vi "BDR_Report.vi"(8 "error in (no error)":errorcluster, 11 "Ref In":T1={"MS SQL Connection"=refnum, "UDL File"=path "", "Time"="", "DCODE"="", "WIP+1"=0, "MC No?"=0, "POKAYOKE?"=FALSE, "Expected Result"="", "Result [Status]"="", "Clock"=0.0, "RFID"="", "WIP Queue"=refnum, "TS Parameter"={"ProfitCenterCode"="", "LineCode"="", "WorkOrderNumber"="", "Model"="", "Model_with_Prefix"="", "VendorCode"="", "SetParameterDateCode"="", "PokaYoke"=0, "Target"=1, "Live_DateCode"="", "CustomerPartNumber"="", "Hand"="", "sBarcode"=FALSE, "FCA"=0, "Ent_Stamp"=timestamp(0 s since 1904-01-01), "STS_CD"=0.0}, "Data_Queue"=[], "RFID Serial No."=""} {"TS Parameter"."FCA" format="%01d"; "TS Parameter"."Target" min=1 max=100000; "TS Parameter"."PokaYoke" min=0 max=1}) -> (0 "error out":errorcluster)   [LabVIEW 2020]
uses:
  Controls/TD SQL.ctl
  <vilib>/addons/database/Connection.llb/Conn ObjectReference.ctl
  Controls/WIP_State.ctl
  Controls/TS_Parameter.ctl
  <vilib>/addons/database/Connection.llb/Conn Execute.vi
  <vilib>/addons/database/Recordset.llb/Rec Fetch Recordset Data (R).vi
  <vilib>/addons/database/Recordset.llb/Rec Destroy - Connection.vi
  <vilib>/addons/database/_DB Variant To Data/Database Variant To Data.xnode
  <vilib>/addons/database/NI_Database_API.lvlib
panel:
  in  "Exit":bool
  in  "Report":i32(listbox)
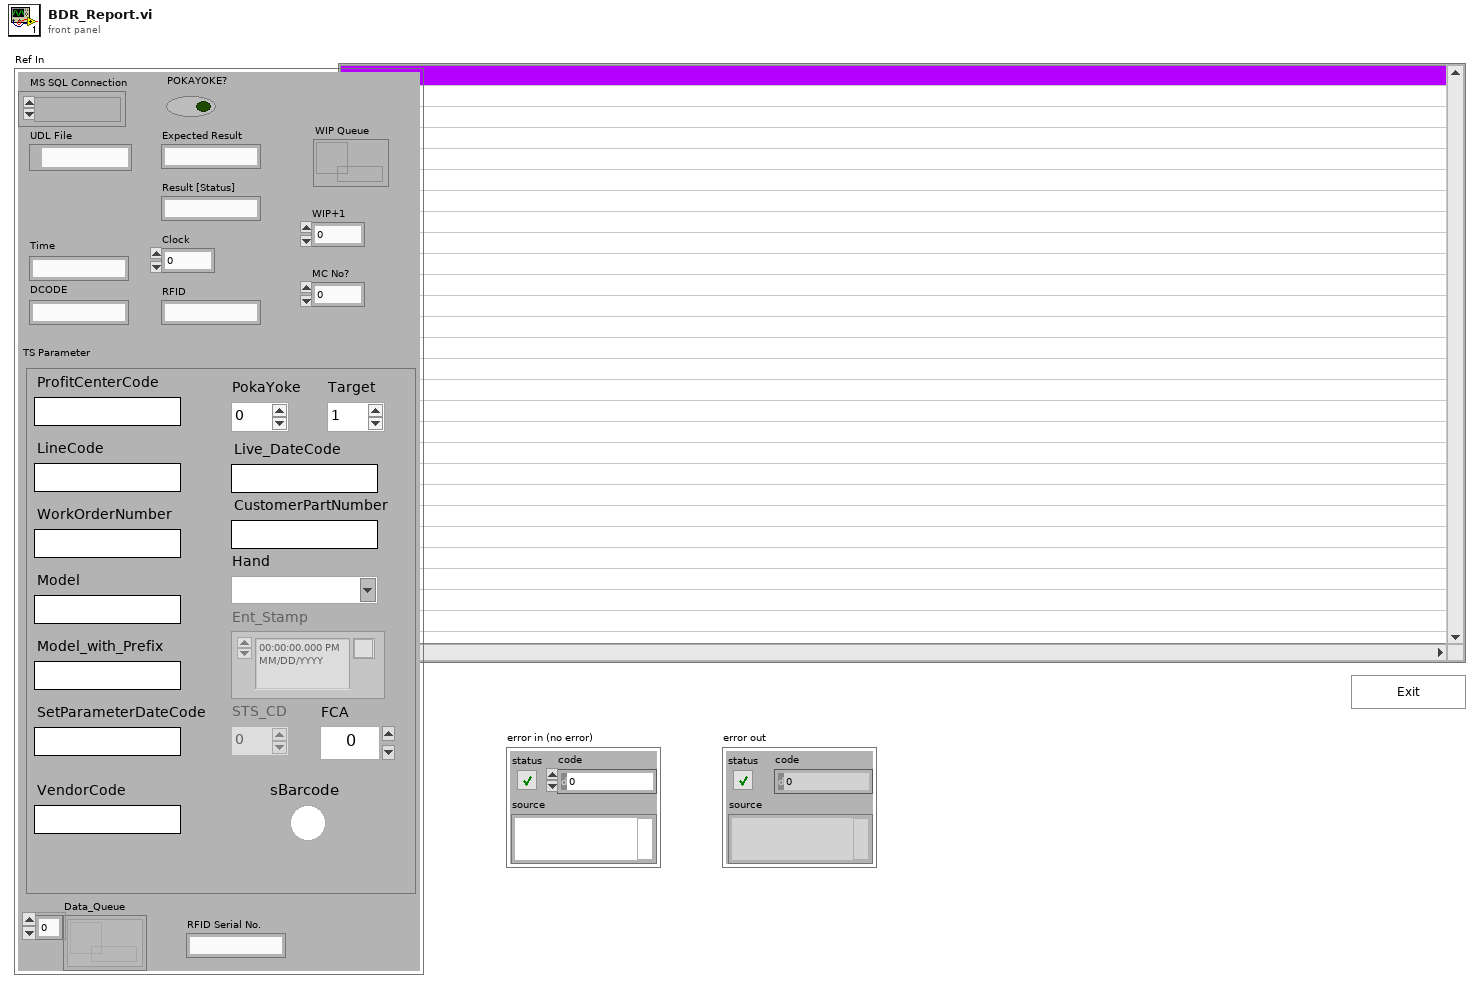
[diagram p1: front panel]
types:
  T1 = typedef "TD SQL.ctl" = cluster{"MS SQL Connection":T2, "UDL File":path, "Time":string, "DCODE":string, "WIP+1":i64, "MC No?":i32, "POKAYOKE?":bool, "Expected Result":string, "Result [Status]":string, "Clock":dbl, "RFID":string, "WIP Queue":refnum<queue>, "TS Parameter":T3, "Data_Queue":refnum<queue>[], "RFID Serial No.":string}
  T2 = typedef "NI_Database_API.lvlib/Conn ObjectReference.ctl" = refnum<k1>
  T3 = typedef "TS_Parameter.ctl" = cluster{"ProfitCenterCode":string, "LineCode":string, "WorkOrderNumber":string, "Model":string, "Model_with_Prefix":string, "VendorCode":string, "SetParameterDateCode":string, "PokaYoke":i32, "Target":i32, "Live_DateCode":string, "CustomerPartNumber":string, "Hand":string, "sBarcode":bool, "FCA":i32, "Ent_Stamp":timestamp, "STS_CD":dbl}
  T4 = typedef "NI_Database_API.lvlib/Rec ObjectReference.ctl" = refnum<k1>
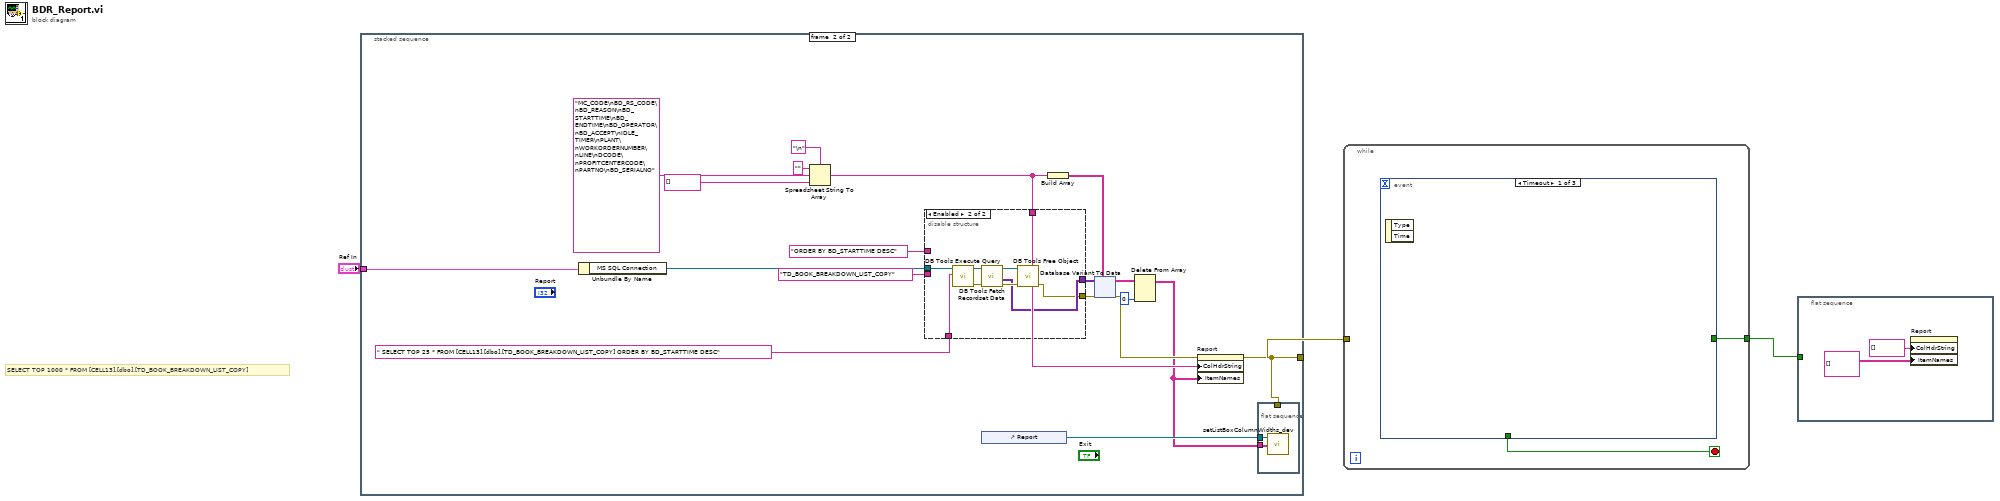
[diagram p0: block diagram]
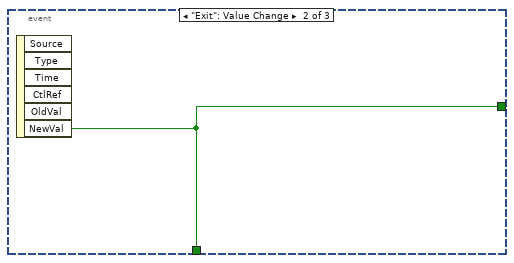
[diagram p2: hidden frame]
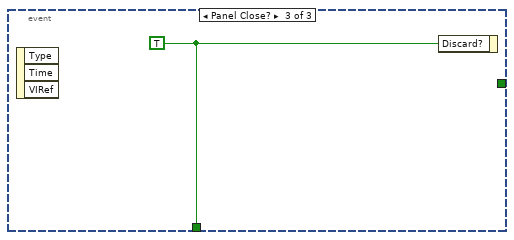
[diagram p3: hidden frame]
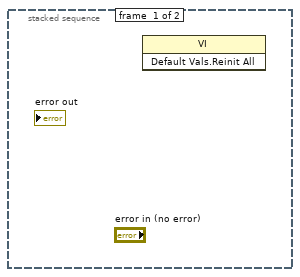
[diagram p4: hidden frame]
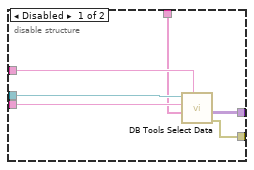
[diagram p5: hidden frame]
diagram:
  # "SELECT TOP 1000 * FROM [CELL13].[dbo].[TD_BOOK_BREAKDOWN_LIST_COPY]"
  n1 = stacked-sequence {
    tunnel: "Ref In" -> [_ w8]
    tunnel: [_ w9] -> w3
    frame #0 {
      n2 = invoke class="VI" method="Default Vals.Reinit All"() -> ()  [unwired: 3 in, 3 out]
    }
    frame #1 {
      n3 = Unbundle By Name(w8) -> ("MS SQL Connection"=w22:T2)
      n4 = Spreadsheet String To Array(delimiter (Tab)="\n", format string="", spreadsheet string="MC_CODE\nBD_RS_CODE\nBD_REASON\nBD_STARTTIME\nBD_ENDTIME\nBD_OPERATOR\nBD_ACCEPT\nIDLE_TIMER\nPLANT\nWORKORDERNUMBER\nLINE\nDCODE\nPROFITCENTERCODE\nPARTNO\nBD_SERIALNO", array type (2D Dbl)=string[] []) -> (array=w13:string[])
      n5 = disable-structure shown="Enabled" {
        disable-tunnel: w22 -> [w28 w32]
        disable-tunnel: "TD_BOOK_BREAKDOWN_LIST_COPY" ("table") -> [w27 _]
        disable-tunnel: [w26 w31] -> w16
        disable-tunnel: "ORDER BY BD_STARTTIME DESC" ("condition") -> [w25 _]
        disable-tunnel: w13 -> [w24 _]
        disable-tunnel: [w23 w29] -> w11
        disable-tunnel: " SELECT TOP 25 * FROM [CELL13].[dbo].[TD_BOOK_BREAKDOWN_LIST_COPY] ORDER BY BD_STARTTIME DESC" ("condition") -> [_ w30]
        frame Disabled {
          n6 = call <vilib>:"DB Tools Select Data.vi"("condition"=w25, "columns"=w24, "table"=w27, "connection reference"=w28) -> ("error out"=w23:errorcluster, "data"=w26:variant[][])  [unwired: 2 in, 1 out]
        }
        frame Enabled {
          n7 = call-poly <vilib>:"DB Tools Execute Query.vi"("SQL query"=w30, "connection reference"=w32) -> ("error out"=w34:errorcluster, "recordset reference"=w35:T4)  [unwired: 6 in]
          n8 = call-poly <vilib>:"DB Tools Fetch Recordset Data.vi"("error in (no error)"=w34, "recordset reference"=w35) -> ("error out"=w33:errorcluster, "recordset data"=w31:variant[][], "recordset reference out"=w36:T4)  [unwired: 3 in]
          n9 = call-poly <vilib>:"DB Tools Free Object.vi"("error in (no error)"=w33, "recordset reference"=w36) -> ("error out"=w29:errorcluster)  [unwired: 8 in, 1 out]
        }
      }
      n10 = control-ref of="Report"() -> (w12:refnum<vi>)
      n11 = Build Array(w13) -> (w15:string[][])
      n12 = xnode "Database Variant To Data"("database variant"=w16, "error in (no error)"=w11, "type"=w15) -> ("data"=w5:string[][], "error out"=w10:errorcluster)
      n13 = Delete From Array(array=w5, index (col)=0 ("disabled index (col)")) -> (array with subset deleted=w6:string[][])  [unwired: 2 in, 1 out]
      n14 = property on="Report" class="MCListbox (strict)"(error in=w10, "ColHdrString"=w13, "ItemNames"=w6) -> (error out=w9:errorcluster)  [unwired: 1 in, 1 out]
      n15 = flat-sequence {
        tunnel: w6 -> [w38]
        tunnel: w12 -> [w37]
        tunnel: w9 -> [_]
        frame #0 {
          n16 = call "setListBoxColumnWidths_dev.vi"("table data"=w38, "MCListbox Refnum"=w37) -> ()  [unwired: 1 in]
        }
      }
    }
  }
  n17 = while {
    tunnel: w3 -> [_]
    tunnel: [w83] -> w1
    stop <- w84 stop-if-true
    n18 = event shown="[0] Timeout" {
      selector: _ -> [_ _ _]
      dyn-events: _ -> [_ _ _]
      timeout: _ -> [_ _ _]
      tunnel: [_ w85 w86] -> w84
      tunnel: [_ w85 _] -> w83
      event Timeout {
        n19 = event-data() -> ()  [unwired: 1 in, 2 out]
      }
      event "Exit": Value Change {
        n20 = event-data() -> ("NewVal"=w85:bool)  [unwired: 1 in, 5 out]
      }
      event Panel Close? {
        w86 = TRUE ("Discard?")
        n21 = event-data() -> ()  [unwired: 1 in, 3 out]
        n22 = event-data("Discard?"=w86) -> ()  [unwired: 1 in, 1 out]
      }
    }
  }
  n23 = flat-sequence {
    tunnel: w1 -> [_]
    frame #0 {
      n24 = property on="Report" class="MCListbox (strict)"("ColHdrString"=string[] [] ("Column Header Strings[]"), "ItemNames"=string[][] [] ("Item Names")) -> ()  [unwired: 2 in, 2 out]
    }
  }
